vi "Filter Control Drag Over Event.vi"(8 "error in (no error)":errorcluster, 10 "ControlDragOverMsg":refnum<class "ControlDragOverMsg.lvclass">, 11 "File Explorer Event Filter in":refnum<class "File Explorer Event Filter.lvclass">) -> (0 "error out":errorcluster, 1 "Discard?":bool, 3 "File Explorer Event Filter out":refnum<class "File Explorer Event Filter.lvclass">)   [LabVIEW 2019, in "File Explorer.lvlib" / "File Explorer Event Filter.lvclass"]
uses:
  <vilib>/gpm_packages/@cs/file-explorer-extension/Source/File Explorer/File Explorer Event Filter/File Explorer Event Filter.lvclass
  <vilib>/gpm_packages/@cs/mva-viewable/Source/ActorEvents/IEventAggregator Messages/ControlDragOverMsg/ControlDragOverMsg.lvclass
  <vilib>/gpm_packages/@cs/mva-viewable/Source/ActorEvents/IEventFilter/IEventFilter.lvclass
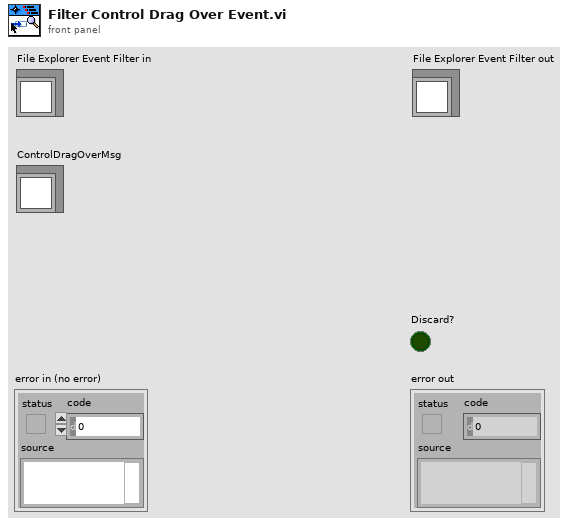
[diagram p1: front panel]
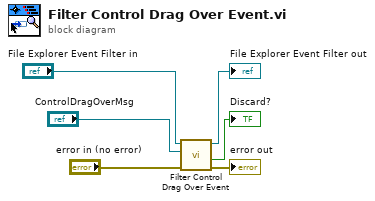
[diagram p0: block diagram]
diagram:
  n1 = call-parent "Filter Control Drag Over Event.vi"("error in (no error)"="error in (no error)", "ControlDragOverMsg"="ControlDragOverMsg", "IEventFilter in"="File Explorer Event Filter in") -> ("error out"=→"error out":errorcluster, "Discard?"=→"Discard?":bool, "IEventFilter out"=→"File Explorer Event Filter out":refnum<class "File Explorer Event Filter.lvclass">)  [unwired: 6 in]
